vi "Oscilloscopio.vi"() -> ()   [LabVIEW 2021]
uses:
  <vilib>/Utility/error.llb/DialogType.ctl
  <instrlib>/Tektronix MSO5X Series/Public/Configure/Configure Trigger (Edge).vi
  <instrlib>/Tektronix MSO5X Series/Public/Data/Read (Single Waveform).vi
  <vilib>/express/express analysis/Spectral/Block/exnSpectralBlock spectral measurements peak poly.vi
  <vilib>/express/express analysis/Spectral/Block/exnSpectralBlock spectral measurements peak WFM.vi
  <vilib>/measure/madcrms.llb/Basic Averaged DC-RMS for 1 Chan.vi
  <vilib>/express/express analysis/Spectral/XNode/ExpressSpectralMeasurementsBlockNode.xnode
  <vilib>/measure/NI_MAPro.lvlib
  <instrlib>/Tektronix MSO5X Series/Tektronix MSO5X Series.lvlib
panel:
  in  "Filename":path=path "test.lvm"
  in  "Enable salvataggi":bool=TRUE caption="Enable"
  in  "Reset misure":bool
  in  "Waveform File":string="TEK00000.WFM"
  in  "Source Channel (CH1)":string="CH1"
  out "Phase":cluster{"f0":dbl, "df":dbl, "phase":dbl[]}
  in  "Saving":bool
  in  "Starting Point (1)":i32=1
  in  "Enable Continuous Acquisition Mode (True)":bool=TRUE caption="Enable Continuous\nAcquisition Mode (True)"
  in  "Vertical Offset (0.0 V)":dbl
  in  "Position (50 %)":dbl=50.0
  out "FFT - (Peak)":cluster{"f0":dbl, "df":dbl, "magnitude":dbl[]}
  in  "Ending Point (2500)":i32=2500
  in  "Slope (0:Rise)":u16(ring) items=["Rise", "Fall", "Either"]
  in  "Trigger Level (0.0V)":dbl
  in  "Vertical Coupling (1: DC)":u16(ring)=1 items=["AC", "DC", "DC Reject"]
  in  "Timebase (40 ns)":dbl=40.0
  in  "Net Attenuation (1.0)":dbl=1.0
  in  "Vertical Range (10.0 V)":dbl=10.0
  in  "Reset":bool
  out "output cluster\n(dati)":T1
  out "appended array\n(array di dati)":dbl[](array[numeric])
  out "Waveform Data":waveform(dbl)(graph)
  in  "VISA Resource Name":refnum<visa-resource-name>="GPIB0::1::INSTR"
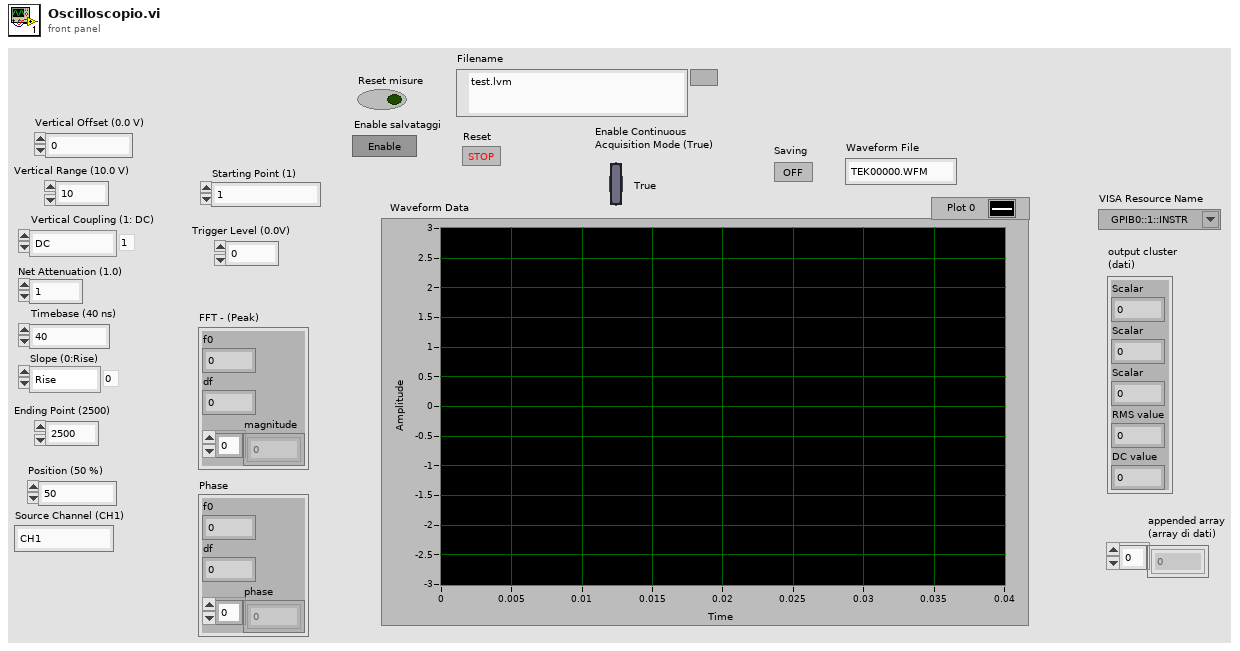
[diagram p1: front panel]
types:
  T1 = cluster{"Scalar":dbl, "Scalar":dbl, "Scalar":dbl, "RMS value":dbl, "DC value":dbl}
  T2 = typedef "DialogType.ctl" = u16
  T3 = enum16{"Rectangular (none)", "Hanning", "Low side lobe"}
  T4 = cluster{"averaging mode":u16, "weighting mode":u16, "number of averages":u32}
  T5 = cluster{"dB On (F)":bool, "unwrap phase (F)":bool, "convert to degree (F)":bool}
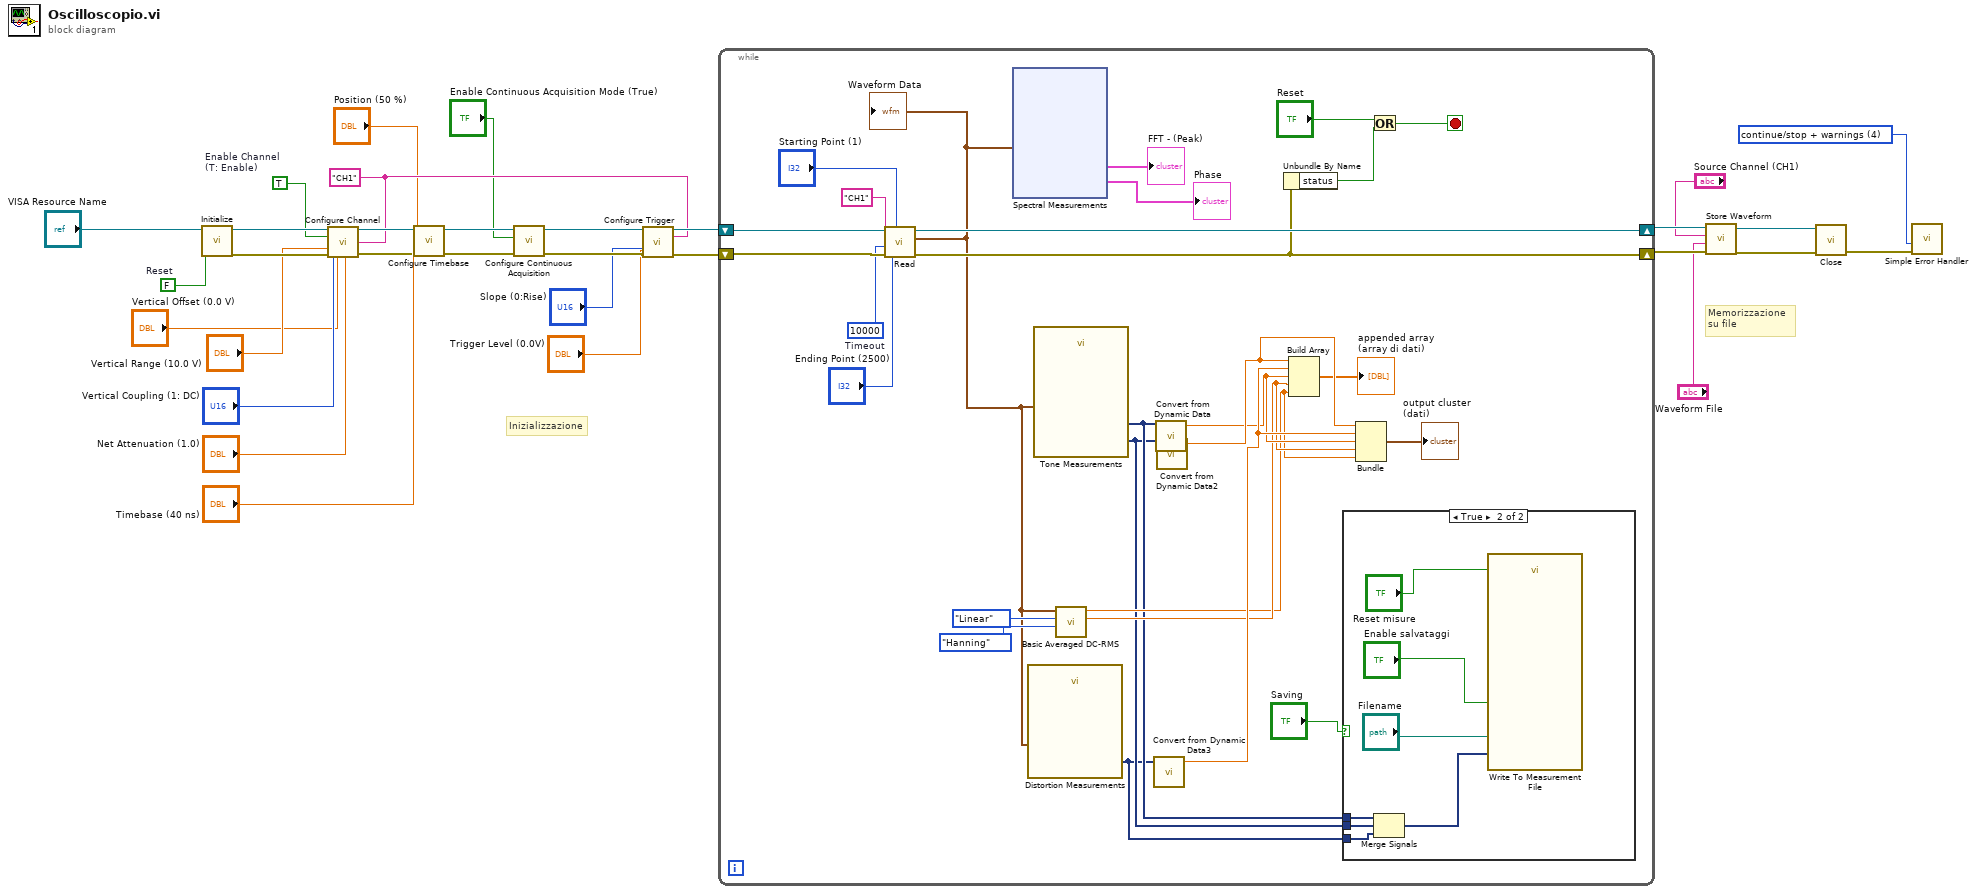
[diagram p0: block diagram]
diagram:
  w11 = "CH1" ("Channel (CH1)")
  w14 = TRUE  # Enable Channel (T: Enable)
  w16 = FALSE  # Reset
  w31 = T2 4 items=["no dialog", "OK message", "continue or stop message", "OK message + warnings", "continue/stop + warnings"] ("type of dialog (OK msg:1)")
  # "Memorizzazione\nsu file"
  # "Inizializzazione"
  n1 = call <instrlib>:"Initialize.vi"("Reset (True)"=w16, "VISA resource name"="VISA Resource Name") -> ("error out"=w17:errorcluster, "VISA resource name out"=w26:refnum<visa-resource-name>)  [unwired: 8 in]
  n2 = call <instrlib>:"Configure Channel.vi"("VISA resource name"=w26, "Vertical Offset (0.0 V)"="Vertical Offset (0.0 V)", "Enable Channel (T: Enable)"=w14, "Channel (CH1)"=w11, "Vertical Range (10.0 V)"="Vertical Range (10.0 V)", "error in (no error)"=w17, "Vertical Coupling (1: DC)"="Vertical Coupling (1: DC)", "Net Attenuation (1.0)"="Net Attenuation (1.0)") -> ("VISA resource name out"=w25:refnum<visa-resource-name>, "error out"=w18:errorcluster)  [unwired: 6 in]
  n3 = call <instrlib>:"Configure Timebase.vi"("error in (no error)"=w18, "Position (50 %)"="Position (50 %)", "Timebase (40 ns)"="Timebase (40 ns)", "VISA resource name"=w25) -> ("error out"=w19:errorcluster, "VISA resource name out"=w24:refnum<visa-resource-name>)  [unwired: 6 in]
  n4 = call <instrlib>:"Configure Continuous Acquisition.vi"("error in (no error)"=w19, "Enable Continuous Acquisition Mode (True)"="Enable Continuous Acquisition Mode (True)", "VISA resource name"=w24) -> ("error out"=w22:errorcluster, "VISA resource name out"=w23:refnum<visa-resource-name>)  [unwired: 7 in]
  n5 = call-poly <instrlib>:"Configure Trigger.vi"("VISA resource name"=w23, "Trigger Source (CH1)"=w11, "Slope (0:Rise)"="Slope (0:Rise)", "error in (no error)"=w22, "Trigger Level (0.0V)"="Trigger Level (0.0V)") -> ("VISA resource name out"=w21:refnum<visa-resource-name>, "error out"=w20:errorcluster)  [unwired: 9 in]
  n6 = while {
    shift-right: [w45] -> w4
    shift-left: w20 -> [w44]
    shift-right: [w46] -> w3
    shift-left: w21 -> [w43]
    stop <- w47 stop-if-true
    w40 = u32 10000  # Timeout
    n7 = call-poly <instrlib>:"Read.vi"("Ending Point (2500)"="Ending Point (2500)", "Starting Point (1)"="Starting Point (1)", "error in (no error)"=w44, "Maximum Time (100000 ms)"=w40, "Channel (CH1)"="CH1", "VISA resource name"=w43) -> ("error out"=w45:errorcluster, "Waveform Graph"=w42:waveform(dbl), "VISA resource name out"=w46:refnum<visa-resource-name>)  [unwired: 3 in]
    "Waveform Data" <- w42
    n8 = xnode "Spectral Measurements"("Signals"=w42) -> ("FFT - (Peak)"=→"FFT - (Peak)":cluster{"f0":dbl, "df":dbl, "magnitude":dbl[]}, "Phase"=→"Phase":cluster{"f0":dbl, "df":dbl, "phase":dbl[]})  [unwired: 1 in, 1 out]
    n9 = call "Distortion Measurements"("Signals"=w42) -> ("THD"=w32:dynamicdata)  [unwired: 9 in, 1 out]
    n10 = call "Tone Measurements"("Signals"=w42) -> ("Frequency"=w35:dynamicdata, "Amplitude"=w36:dynamicdata)  [unwired: 8 in, 1 out]
    n11 = call-poly <vilib>:"Basic Averaged DC-RMS.vi"("window"=T3."Hanning", "averaging type"=enum16{"Linear", "Exponential"}."Linear", "signal in"=w42) -> ("RMS value"=w53:dbl, "DC value"=w52:dbl)  [unwired: 5 in, 2 out]
    n12 = call "Convert from Dynamic Data3"("Dynamic Data Type"=w32) -> ("Scalar"=w55:dbl)  [unwired: 3 in]
    n13 = call "Convert from Dynamic Data"("Dynamic Data Type"=w36) -> ("Scalar"=w54:dbl)  [unwired: 3 in]
    n14 = call "Convert from Dynamic Data2"("Dynamic Data Type"=w35) -> ("Scalar"=w56:dbl)  [unwired: 3 in]
    n15 = Unbundle By Name(w45) -> ("status"=w49:bool)
    n16 = Build Array "Build Array"(w56, w55, w54, w53, w52) -> (→"appended array\n(array di dati)":dbl[])
    n17 = case shown="True" "Saving" {
      tunnel: w36 -> [_ w65]
      tunnel: w35 -> [_ w64]
      tunnel: w32 -> [_ w60]
      frame False {
      }
      frame True {
        n18 = Merge Signals(w65, w64, w60) -> (w63:dynamicdata)
        n19 = call "Write To Measurement File"("Signals"=w63, "Reset"="Reset misure", "Enable"="Enable salvataggi", "Filename"="Filename") -> ()  [unwired: 13 in, 3 out]
      }
    }
    n20 = Bundle("Scalar"=w56, "Scalar"=w55, "Scalar"=w54, "RMS value"=w53, "DC value"=w52) -> (→"output cluster\n(dati)":T1)  [unwired: 1 in]
    n21 = Or(x="Reset", y=w49) -> (x .or. y?=w47:bool)
  }
  n22 = call <instrlib>:"Store Waveform.vi"("error in (no error)"=w4, "Waveform File"="Waveform File", "Source Channel (CH1)"="Source Channel (CH1)", "VISA resource name"=w3) -> ("error out"=w5:errorcluster, "VISA resource name out"=w6:refnum<visa-resource-name>)  [unwired: 6 in]
  n23 = call <instrlib>:"Close.vi"("error in (no error)"=w5, "VISA resource name"=w6) -> ("error out"=w7:errorcluster)  [unwired: 9 in]
  n24 = call <vilib>:"Simple Error Handler.vi"("type of dialog (OK msg:1)"=w31, "error in (no error)"=w7) -> ()  [unwired: 3 in, 5 out]
